vi "Write Data.vi"(9 "Trial Results":string[](array[string]), 11 "base path":path) -> ()   [LabVIEW 2013]
uses:
  <vilib>/Utility/file.llb/Write To Spreadsheet File (string).vi
panel:
  in  "Case Constant\n(See Context Help)":bool
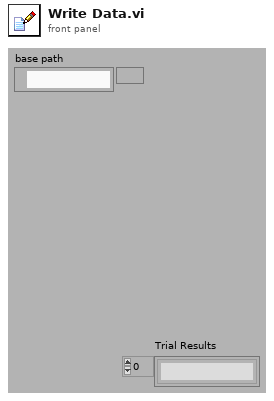
[diagram p1: front panel]
types:
  T1 = enum16{"open", "open or create", "create or replace", "create", "open (read only)"}
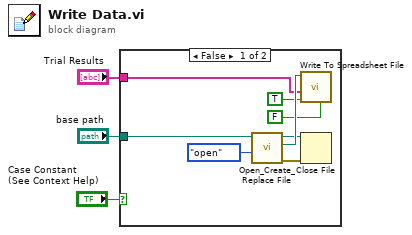
[diagram p0: block diagram]
diagram:
  n1 = case shown="False" "Case Constant\n(See Context Help)" {
    tunnel: "base path" -> [w10 _]
    tunnel: "Trial Results" -> [w4 _]
    frame False {
      n2 = call <vilib>:"Open_Create_Replace File.vi"("function (open:0)"=T1."open", "file path"=w10) -> ("error out"=w6:errorcluster, "new file path"=w9:path, "refnum"=w7:refnum<file>)  [unwired: 6 in, 1 out]
      n3 = call-poly <vilib>:"Write To Spreadsheet File.vi"("transpose? (no:F)"=FALSE, "append to file? (new file:F)"=TRUE, "1D data"=w4, "file path (dialog if empty)"=w9) -> ()  [unwired: 4 in, 1 out]
      n4 = Close File(refnum=w7, error in=w6) -> ()  [unwired: 2 out]
    }
    frame True {
    }
  }
